vi "Read Alive_.vi"(8 "error in (no error)":errorcluster, 11 "PlayerUpdate in":refnum<class "PlayerUpdate.lvclass">) -> (0 "error out":errorcluster, 2 "Alive?":bool, 3 "PlayerUpdate out":refnum<class "PlayerUpdate.lvclass">)   [LabVIEW 2019, in "PlayerUpdate.lvclass"]
uses:
  PlayerUpdate.lvclass
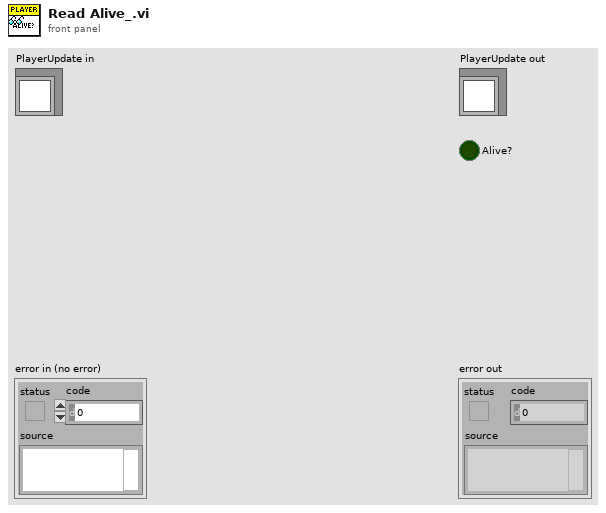
[diagram p1: front panel]
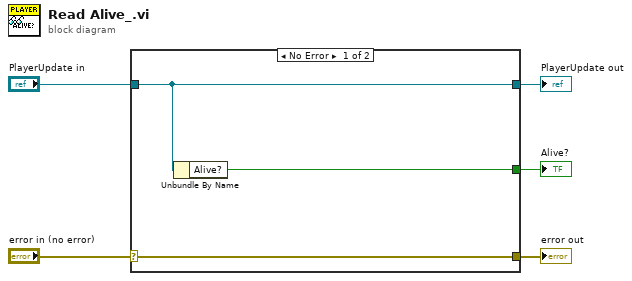
[diagram p0: block diagram]
diagram:
  n1 = case shown="No Error" "error in (no error)" {
    selector: "error in (no error)" -> [w8 w9]
    tunnel: [w8 w9] -> w4
    tunnel: [w7 w10] -> w2
    tunnel: "PlayerUpdate in" -> [w7 w10]
    tunnel: [w6 _] -> w1
    frame No Error {
      n2 = Unbundle By Name(w7) -> ("Alive?"=w6:bool)
    }
    frame Error {
    }
  }
  "error out" <- w4
  "PlayerUpdate out" <- w2
  "Alive?" <- w1
